vi "AddDescriptionToClassPropAccessors.vi"   [LabVIEW 2020]
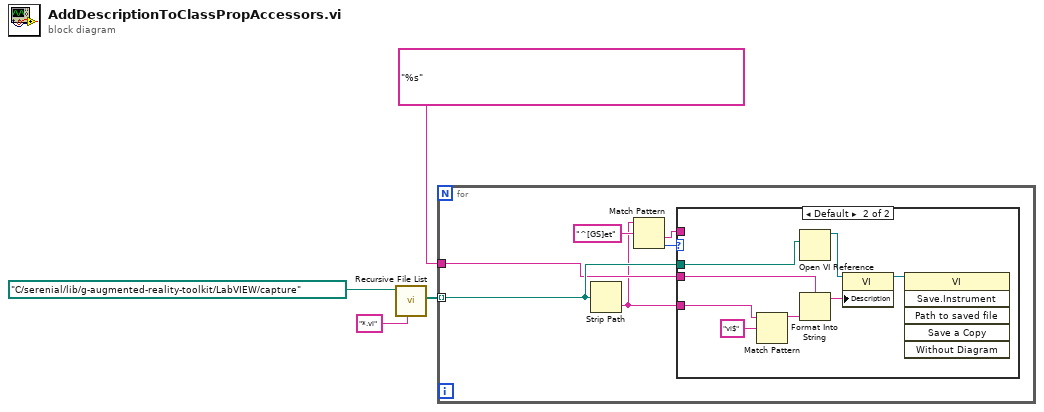
[diagram p0: block diagram]
diagram:
  n1 = call <vilib>:"Recursive File List.vi"("pattern"="*.vi", "Folder Path"=path "C:/serenial/lib/g-augmented-reality-toolkit/LabVIEW/capture") -> ("All Files in Dir"=w3:path[])  [unwired: 5 in, 4 out]
  n2 = for {
    tunnel: w3 -> [w8] mode=indexing
    tunnel: "%s" ("format string") -> [w6]
    n3 = Strip Path(path=w8) -> (name=w5:string)  [unwired: 1 out]
    n4 = Match Pattern(string=w5, regular expression="^[GS]et") -> (after substring=w7:string, offset past match=w9:i32)  [unwired: 1 in, 2 out]
    n5 = case shown="Default" w9 {
      tunnel: w8 -> [_ w18]
      tunnel: w7 -> [_ _]
      tunnel: w6 -> [_ w13]
      tunnel: w5 -> [_ w12]
      frame -1 {
      }
      frame Default {
        n6 = Match Pattern(string=w12, regular expression="vi$") -> (before substring=w11:string)  [unwired: 1 in, 3 out]
        n7 = Open VI Reference(vi path=w18) -> (vi reference=w16:refnum<vi>)  [unwired: 5 in, 1 out]
        n8 = Format Into String(format string=w13, w11) -> (resulting string=w15:string)  [unwired: 2 in, 1 out]
        n9 = property class="VI"(reference=w16, "Description"=w15) -> (reference out=w14:refnum<vi>)  [unwired: 1 in, 1 out]
        n10 = invoke class="VI" method="Save.Instrument"(reference=w14) -> ()  [unwired: 5 in, 6 out]
      }
    }
  }
